vi "Get OOB gRPC Port.vi"(8 "error in (no error)":errorcluster) -> (0 "error out":errorcluster, 3 "OOB gRPC Port":i32)   [LabVIEW 2025, in "I2C Bus Monitor.lvclass"]
uses:
  I2C Bus Monitor.lvclass
  I2C Bus Monitor.lvclass/I2C Bus Monitor.ctl
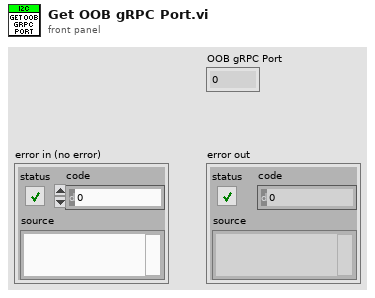
[diagram p1: front panel]
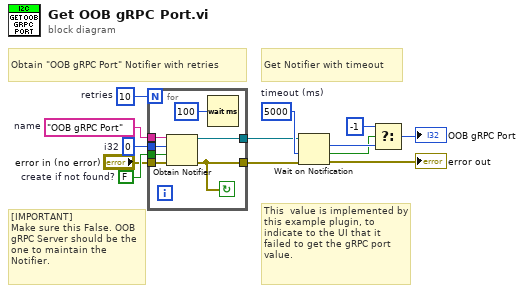
[diagram p0: block diagram]
diagram:
  w13 = FALSE  # create if not found?
  w5 = 0  # i32
  w7 = "OOB gRPC Port"  # name
  w4 = 10  # retries
  w3 = 5000  # timeout (ms)
  # "This  value is implemented by this example plugin, to indicate to the UI that it failed to get the gRPC port value."
  # "[IMPORTANT] \nMake sure this False. OOB gRPC Server should be the one to maintain the Notifier."
  # "Obtain \"OOB gRPC Port\" Notifier with retries"
  # "Get Notifier with timeout"
  n1 = for {
    N: w4 -> [_]
    tunnel: [w18] -> w1
    tunnel: [w20] -> w2
    tunnel: w7 -> [w17]
    tunnel: w5 -> [w16]
    tunnel: "error in (no error)" -> [w15]
    tunnel: w13 -> [w14]
    stop <- w18 continue-if-true
    n2 = Obtain Notifier(name (unnamed)=w17, notification data type=w16, create if not found? (T)=w14, error in (no error)=w15) -> (notifier out=w20:refnum<notifier>, error out=w18:errorcluster)  [unwired: 1 out]
    n3 = Wait (ms)(milliseconds to wait=u32 100) -> ()  [unwired: 1 out]
  }
  n4 = Wait on Notification(notifier=w2, timeout in ms (-1)=w3, error in (no error)=w1) -> (notification=w11:i32, timed out?=w10:bool, error out=→"error out":errorcluster)  [unwired: 1 in, 1 out]
  n5 = Select(t=-1, s=w10, f=w11) -> (s? t:f=→"OOB gRPC Port":i32)
